vi "startup.vi"(8 "error in (no error)":errorcluster, 11 "AnalysisResultsViewer in":refnum<class "AnalysisResultsViewer.lvclass">) -> (0 "error out":errorcluster, 3 "AnalysisResultsViewer out":refnum<class "AnalysisResultsViewer.lvclass">)   [LabVIEW 2009, in "Views.lvlib" / "Camera.lvlib" / "AnalysisResultsViewer.lvclass"]
uses:
  AnalysisResultsViewer.lvclass
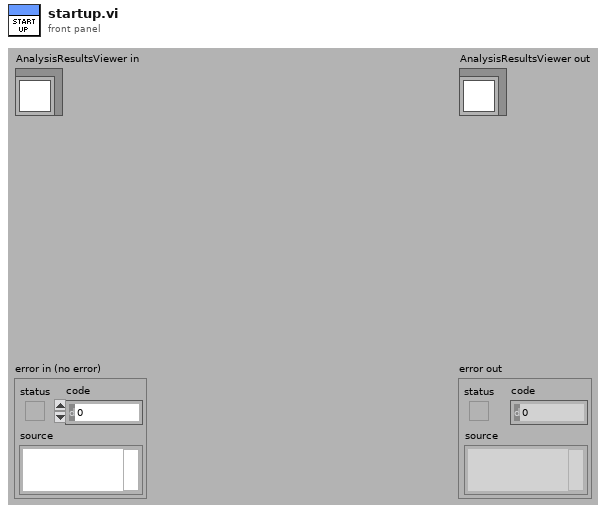
[diagram p1: front panel]
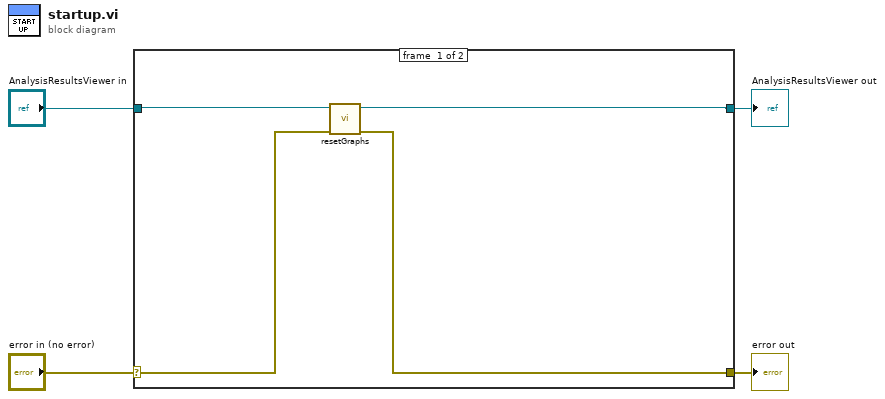
[diagram p0: block diagram]
diagram:
  n1 = case shown="No Error" "error in (no error)" {
    selector: "error in (no error)" -> [w6 w10]
    tunnel: [w5 w10] -> w3
    tunnel: [w7 w9] -> w1
    tunnel: "AnalysisResultsViewer in" -> [w8 w9]
    frame #0 {
      n2 = call "resetGraphs.vi"("error in (no error)"=w6, "AnalysisResultsViewer in"=w8) -> ("error out"=w5:errorcluster, "AnalysisResultsViewer out"=w7:refnum<class "AnalysisResultsViewer.lvclass">)  [unwired: 8 in]
    }
    frame #1 {
    }
  }
  "error out" <- w3
  "AnalysisResultsViewer out" <- w1
